vi "Generate pixels ramp.vi"(1 "DX":i16, 2 "X0":i16) -> (0 "Ramp":i16[](array[numeric]))   [LabVIEW 2009]
uses:
  <vilib>/Analysis/NI_AALBase.lvlib
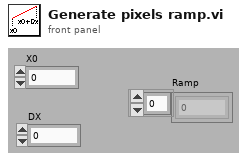
[diagram p1: front panel]
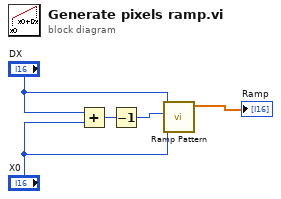
[diagram p0: block diagram]
diagram:
  n1 = Add(x="DX", y="X0") -> (x+y=w3:i16)
  n2 = Decrement(x=w3) -> (x-1=w5:i16)
  n3 = call <vilib>:"Ramp Pattern.vi"("start"="X0", "end"=w5, "samples"="DX") -> ("Ramp Pattern"=→"Ramp":dbl[])  [unwired: 7 in, 1 out]
